vi "SGSA_Sweep.vi"() -> ()   [LabVIEW 2023, in "SG_SA.lvlib"]
uses:
  SG_SA.lvlib
  Clover_Cell.lvlib
panel:
  in  "FileNote":string
  in  "TRXmode":u16(ring)=1 items=["QUERY_TELEM_2 (V)"=2, "QUERY_TELEM_1 (H)"=1]
  in  "AiP_Channe_index":i32(ring) items=["1", "2", "3", "4"]
  in  "AiP_No.":i32(ring) items=["AiP_1", "AiP_2", "AiP_3", "AiP_4", "AiP_5", "AiP_6", "AiP_7", "AiP_8"]
  out "SG Power":i32
  in  "Stop Power":i32=8
  in  "Start Power":i32=-40
  in  "SG":refnum<visa-resource-name>="TCPIP::192.168.100.200::inst0::INSTR"
  in  "AvgTimes":i32=10
  in  "SA":refnum<visa-resource-name>="TCPIP::192.168.100.230::inst0::INSTR"
  # "56"
  # "55"
  # "54"
  # "53"
  # "52"
  # "51"
  # "50"
  # "49"
  # "40"
  # "39"
  # "38"
  # "37"
  # "36"
  # "35"
  # "34"
  # "33"
  # "24"
  # "23"
  # "22"
  # "21"
  # "20"
  # "19"
  # "18"
  # "17"
  # "8"
  # "7"
  # "6"
  # "5"
  # "4"
  # "3"
  # "2"
  # "1"
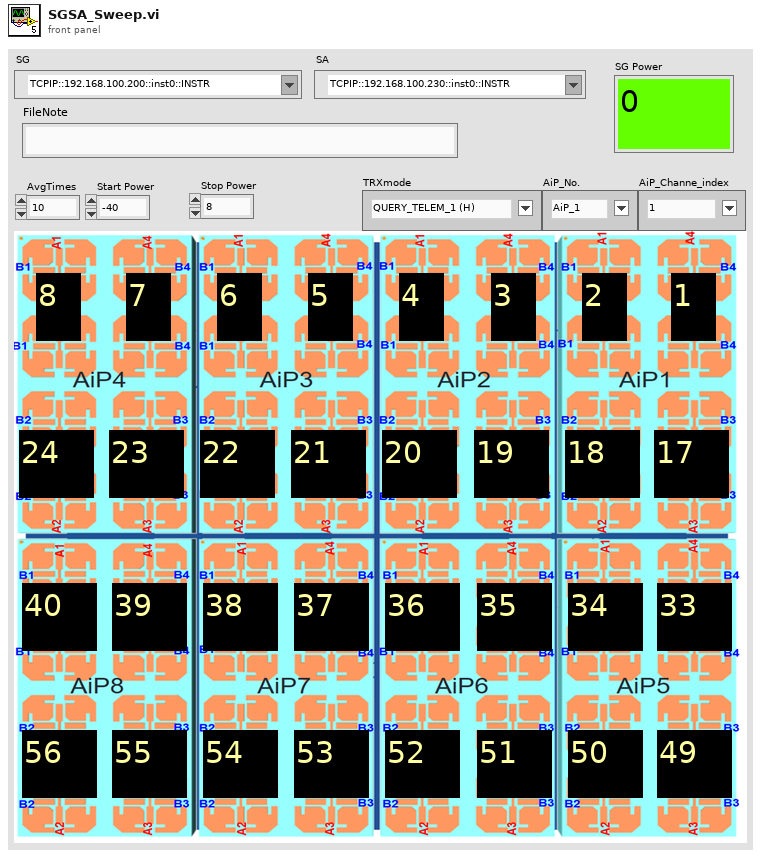
[diagram p1: front panel]
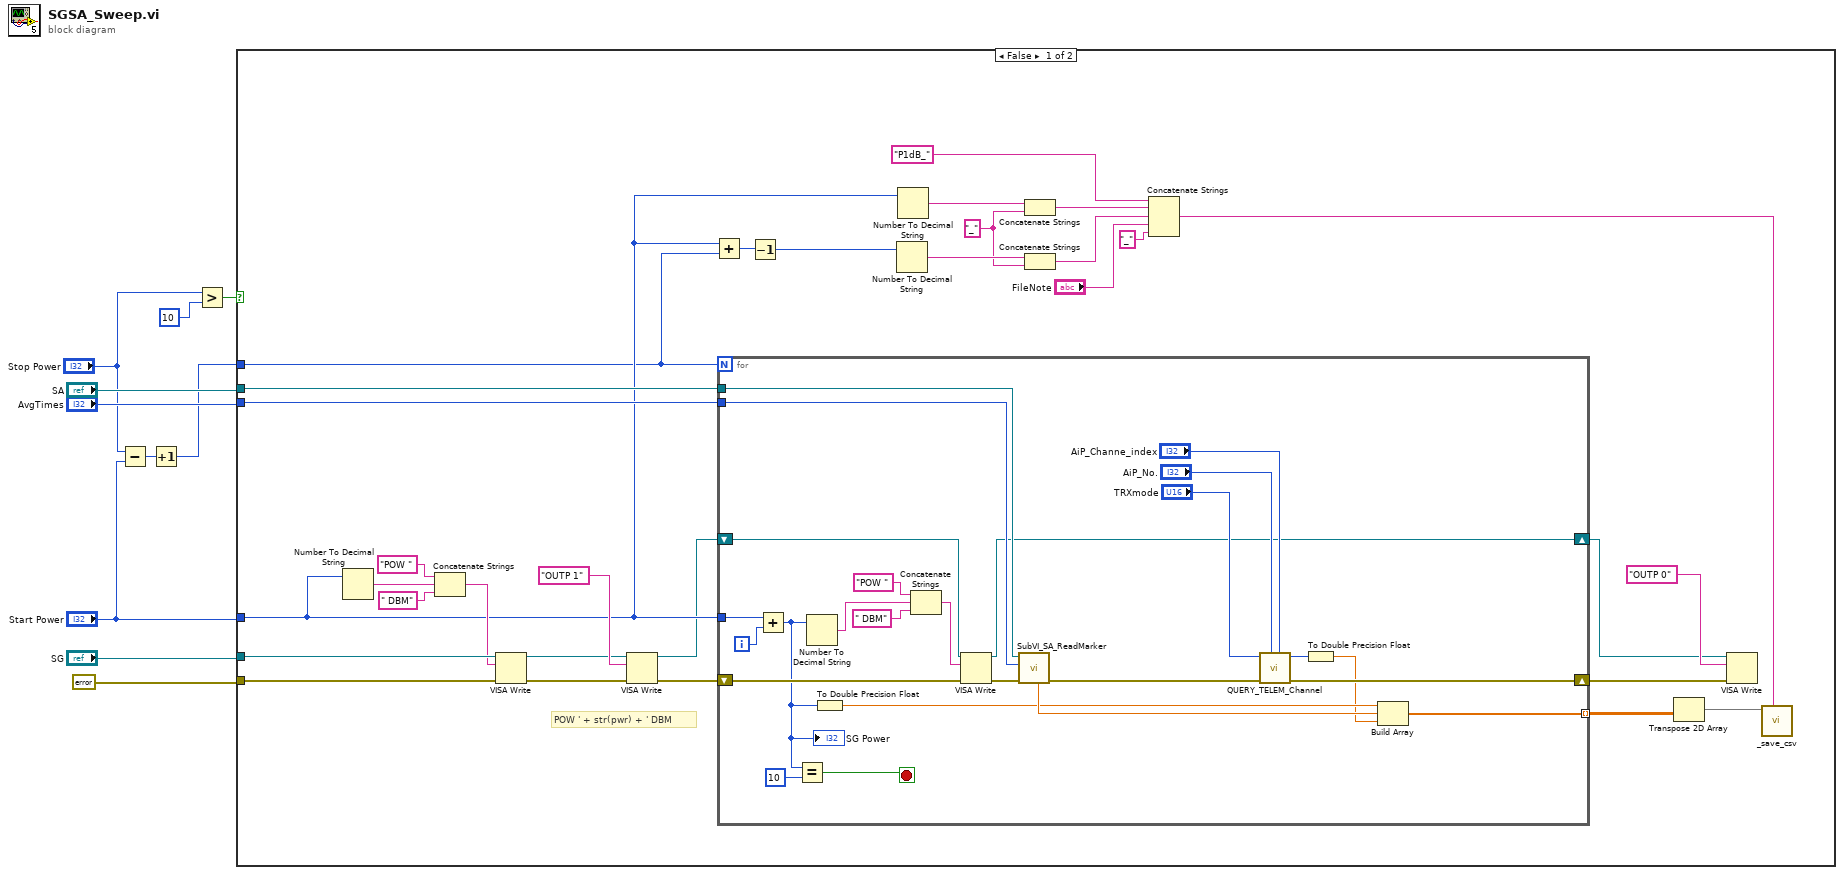
[diagram p0: block diagram]
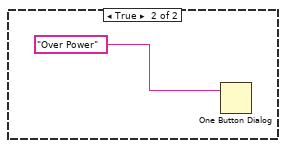
[diagram p2: hidden frame]
diagram:
  n1 = Subtract(x="Stop Power", y="Start Power") -> (x-y=w4:i32)
  n2 = Increment(x=w4) -> (x+1=w3:i32)
  n3 = Greater?(x="Stop Power", y=10) -> (0:w7:bool)
  n4 = case shown="False" w7 {
    tunnel: "SA" -> [w41 _]
    tunnel: "AvgTimes" -> [w40 _]
    tunnel: "Start Power" -> [w16 _]
    tunnel: errorcluster {"status"=FALSE, "code"=0, "source"=""} ("error in (no error)") -> [w20 _]
    tunnel: "SG" -> [w19 _]
    tunnel: w3 -> [w15 _]
    frame False {
      w29 = "_"
      # "POW ' + str(pwr) + ' DBM"
      n5 = Number To Decimal String(number=w16) -> (decimal integer string=w22:string)  [unwired: 1 in]
      n6 = Concatenate Strings("POW ", w22, " DBM") -> (w17:string)
      n7 = VISA Write(VISA resource name=w19, write buffer=w17, error in (no error)=w20) -> (VISA resource name out=w18:refnum<visa-resource-name>, error out=w21:errorcluster)  [unwired: 1 out]
      n8 = VISA Write(VISA resource name=w18, write buffer="OUTP 1", error in (no error)=w21) -> (VISA resource name out=w14:refnum<visa-resource-name>, error out=w37:errorcluster)  [unwired: 1 out]
      n9 = Add(x=w16, y=w15) -> (x+y=w33:i32)
      n10 = for {
        N: w15 -> [_]
        tunnel: w41 -> [w66]
        tunnel: w40 -> [w65]
        tunnel: w16 -> [w61]
        tunnel: [w54] -> w39 mode=indexing
        shift-right: [w49] -> w34
        shift-left: w37 -> [w63]
        shift-right: [w43] -> w13
        shift-left: w14 -> [w42]
        i -> [w62]
        stop <- w51 stop-if-true
        n11 = Add(x=w61, y=w62) -> (x+y=w53:i32)
        "SG Power" <- w53
        n12 = Equal?(x=w53, y=10) -> (x = y?=w51:bool)
        n13 = Number To Decimal String(number=w53) -> (decimal integer string=w58:string)  [unwired: 1 in]
        n14 = To Double Precision Float(number=w53) -> (double precision float=w55:dbl)
        n15 = Concatenate Strings("POW ", w58, " DBM") -> (w57:string)
        n16 = VISA Write(VISA resource name=w42, write buffer=w57, error in (no error)=w63) -> (VISA resource name out=w43:refnum<visa-resource-name>, error out=w64:errorcluster)  [unwired: 1 out]
        n17 = call "SubVI_SA_ReadMarker.vi"("error in (no error)"=w64, "AvgTimes"=w65, "VISA resource name"=w66) -> ("error out"=w50:errorcluster, "Marker Power"=w56:dbl)  [unwired: 5 in, 2 out]
        n18 = call "QUERY_TELEM_Channel.vi"("AiP_ele."="AiP_Channe_index", "AiP_No."="AiP_No.", "error in"=w50, "TRXmode"="TRXmode") -> ("error out"=w49:errorcluster, "pdet"=w46:i32)  [unwired: 6 in]
        n19 = To Double Precision Float(number=w46) -> (double precision float=w45:dbl)
        n20 = Build Array(w55, w56, w45) -> (w54:dbl[])
      }
      n21 = Decrement(x=w33) -> (x-1=w32:i32)
      n22 = Number To Decimal String(number=w32) -> (decimal integer string=w30:string)  [unwired: 1 in]
      n23 = Number To Decimal String(number=w16) -> (decimal integer string=w31:string)  [unwired: 1 in]
      n24 = Concatenate Strings(w31, w29) -> (w27:string)
      n25 = Concatenate Strings(w30, w29) -> (w26:string)
      n26 = Concatenate Strings("P1dB_" ("delimiter (\\t)"), w27, w26, "FileNote", "_") -> (w25:string)
      n27 = Transpose 2D Array(2D array=w39) -> (transposed array=w38:dbl[][])
      n28 = VISA Write(VISA resource name=w13, write buffer="OUTP 0", error in (no error)=w34) -> ()  [unwired: 3 out]
      n29 = call "_save_csv.vi"("delimiter (\\t)"=w25, "Data"=w38) -> ()  [unwired: 9 in, 1 out]
    }
    frame True {
      n30 = One Button Dialog(message="Over Power") -> ()  [unwired: 1 in, 1 out]
    }
  }
